vi "Write basePath.vi"(8 "error in (no error)":errorcluster, 10 "basePath":path, 11 "PolymorphicStructure in":refnum<class "PolymorphicStructure.lvclass">) -> (0 "error out":errorcluster, 3 "PolymorphicStructure out":refnum<class "PolymorphicStructure.lvclass">)   [LabVIEW 2013, in "PolymorphicStructure.lvclass"]
uses:
  PolymorphicStructure.lvclass
  PolymorphicStructure.lvclass/PolymorphicStructure.ctl
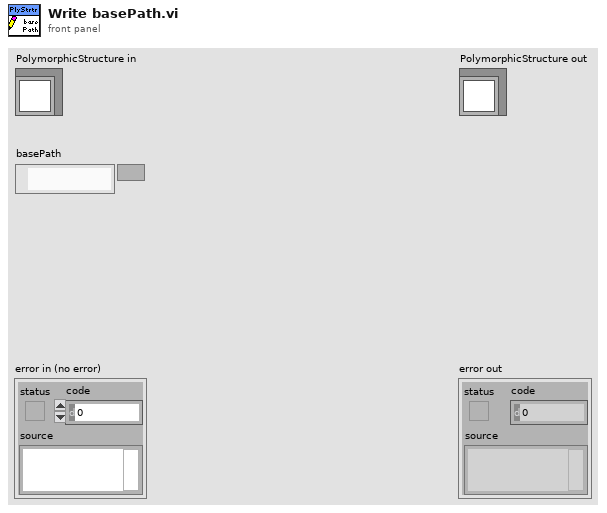
[diagram p1: front panel]
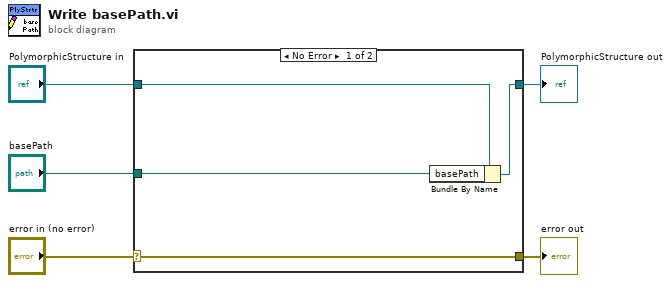
[diagram p0: block diagram]
diagram:
  n1 = case shown="No Error" "error in (no error)" {
    selector: "error in (no error)" -> [w9 w10]
    tunnel: [w9 w10] -> w4
    tunnel: [w7 w11] -> w2
    tunnel: "PolymorphicStructure in" -> [w8 w11]
    tunnel: "basePath" -> [w6 _]
    frame No Error {
      n2 = Bundle By Name(cluster=w8, "basePath"=w6) -> (w7:refnum<class "PolymorphicStructure.lvclass">)
    }
    frame Error {
    }
  }
  "error out" <- w4
  "PolymorphicStructure out" <- w2
